vi "RX — NIRs.vi"() -> ()   [LabVIEW 2020]
panel:
  out "qC/N0":dbl[](array[numeric])
  out "Numeric":dbl
  out "Порог":dbl
  in  "Pлт":dbl=0.0001
  out "Array":cdb[][](array[numeric])
  out "Блок считывания":cdb[][](array[numeric])
  out "qC/N0 dB":dbl[](array[numeric])
  in  "Частота \nдискритезации":dbl=5000000.0 format="%#_13g"
  in  "Время \nнакопления":dbl=0.008 format="%#_13g"
  out "qC/N0":dbl
  out "dopEst":dbl
  out "codePhase":dbl
  in  "Целое число строк записанного файла":i32=50
  in  "Путь к записи сигнала":path=path "C:/Users/ira_1/OneDrive/Рабочий стол/samples.bin"
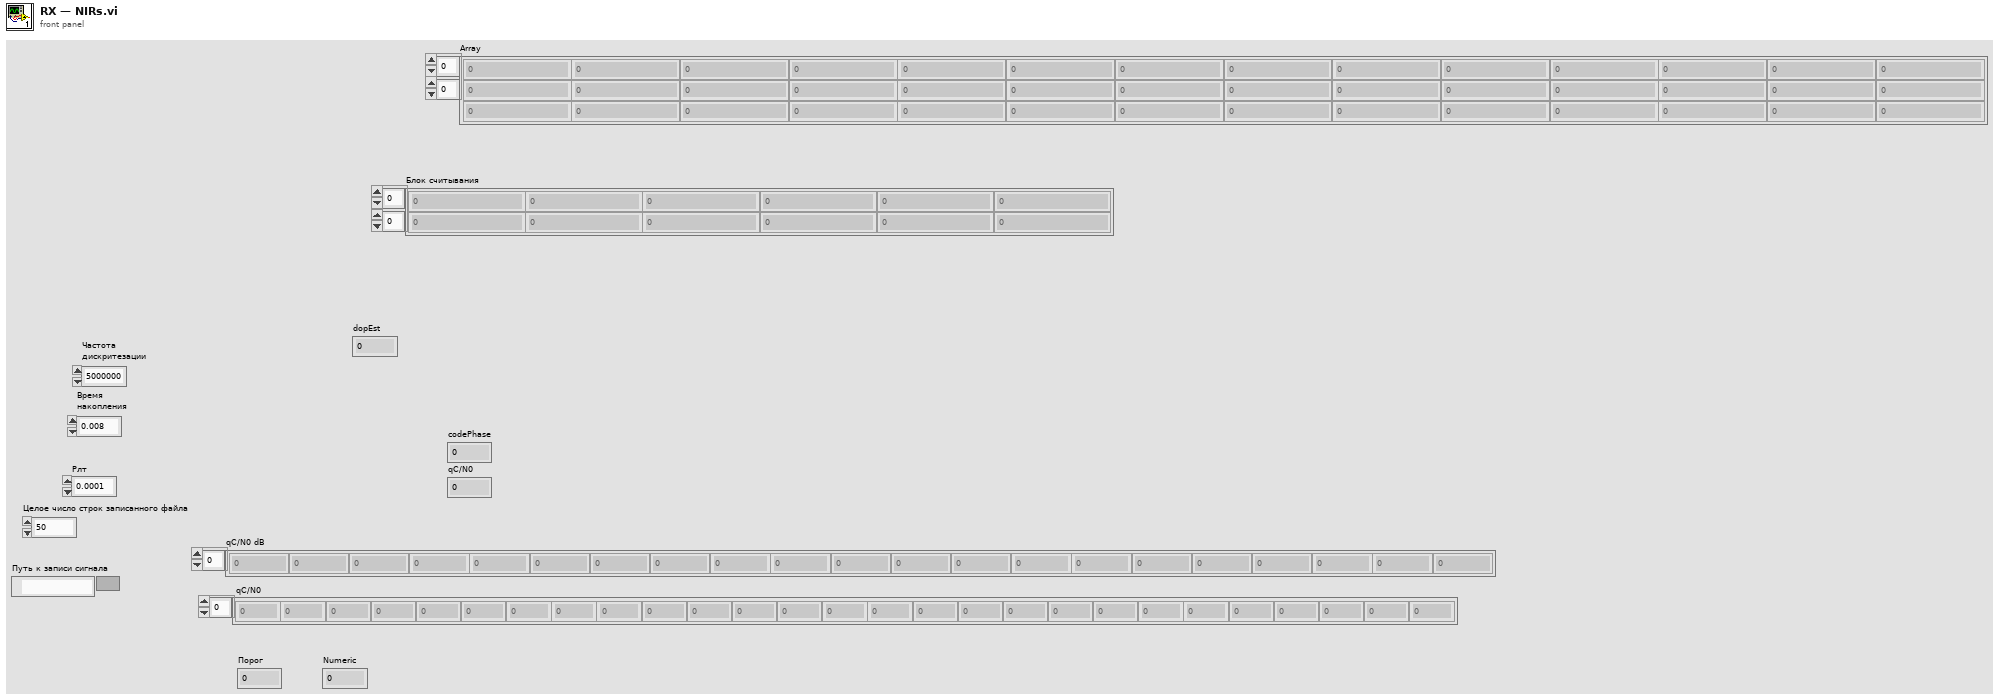
[diagram p1: front panel]
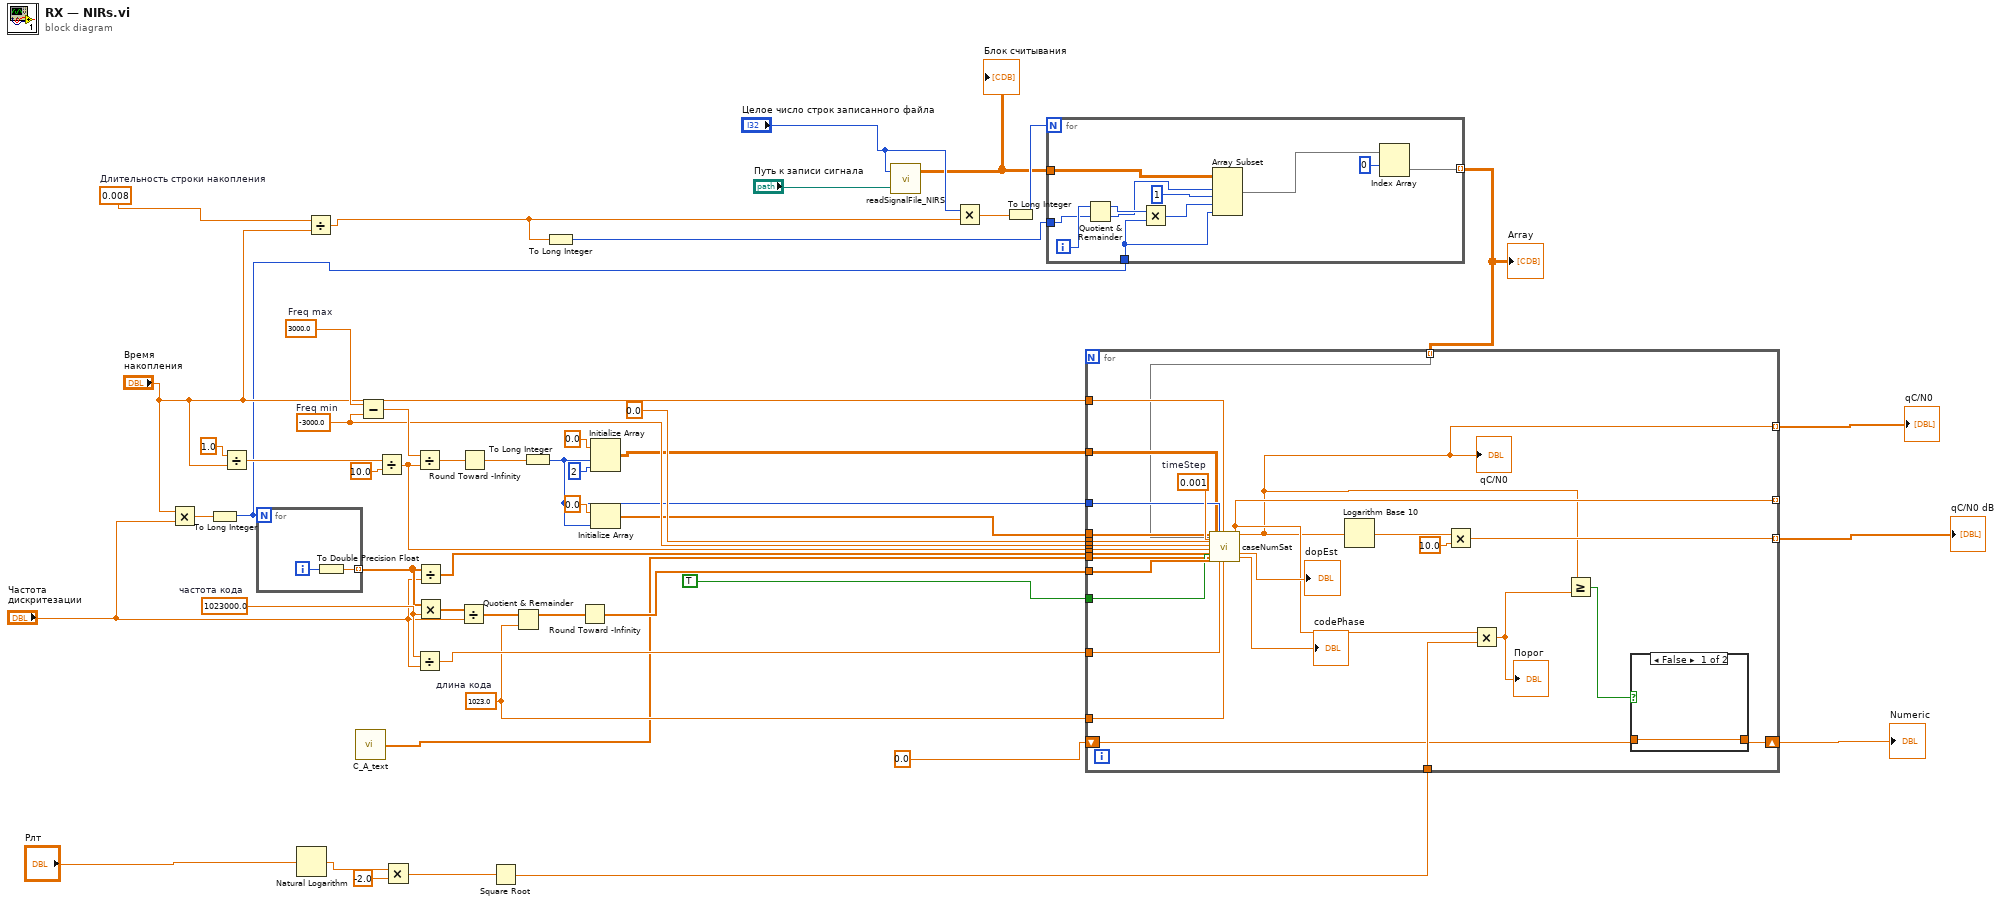
[diagram p0: block diagram]
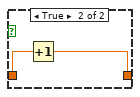
[diagram p2: hidden frame]
diagram:
  w20 = 0.008  # Длительность строки накопления
  w37 = -3000.0  # Freq min
  w43 = 3000.0  # Freq max
  w33 = 1023.0  # длина кода
  w35 = 1023000.0  # частота кода
  n1 = Multiply(x="Время \nнакопления", y="Частота \nдискритезации") -> (x*y=w21:dbl)
  n2 = To Long Integer(number=w21) -> (32bit integer=w14:i32)
  n3 = Divide(x=1.0, y="Время \nнакопления") -> (x/y=w39:dbl)
  n4 = for {
    N: w14 -> [_]
    tunnel: [w50] -> w25 mode=indexing
    i -> [w51]
    n5 = To Double Precision Float(number=w51) -> (double precision float=w50:dbl)
  }
  n6 = Natural Logarithm(1:"Pлт") -> (0:w11:dbl)
  n7 = Divide(x=w20, y="Время \nнакопления") -> (x/y=w16:dbl)
  n8 = call "C_A_text.vi"() -> ("array"=w23:dbl[])  [unwired: 2 in]
  n9 = Subtract(x=w43, y=w37) -> (x-y=w41:dbl)
  n10 = Divide(x=w39, y=10.0) -> (x/y=w36:dbl)
  n11 = Multiply(x=w11, y=-2.0) -> (x*y=w9:dbl)
  n12 = Divide(x=w41, y=w36) -> (x/y=w42:dbl)
  n13 = Divide(x=w35, y="Частота \nдискритезации") -> (x/y=w34:dbl)
  n14 = Divide(x=w25, y="Частота \nдискритезации") -> (x/y=w24:dbl[])
  n15 = Multiply(x=w25, y=w35) -> (x*y=w49:dbl[])
  n16 = Divide(x=w49, y="Частота \nдискритезации") -> (x/y=w48:dbl[])
  n17 = Round Toward -Infinity(1:w42) -> (0:w40:dbl)
  n18 = Square Root(x=w9) -> (sqrt(x)=w7:dbl)
  n19 = Quotient & Remainder(x=w48, y=w33) -> (x-y*floor(x/y)=w47:dbl[])  [unwired: 1 out]
  n20 = To Long Integer(number=w40) -> (32bit integer=w28:i32)
  n21 = To Long Integer(number=w16) -> (32bit integer=w15:i32)
  n22 = Round Toward -Infinity(1:w47) -> (0:w46:dbl[])
  n23 = Initialize Array(0.0 ("element"), w28, 2 ("dimension size")) -> (w27:dbl[][])
  n24 = Initialize Array(0.0 ("element"), w28) -> (w26:dbl[])
  n25 = call "readSignalFile_NIRS.vi"("Путь к записи сигнала"="Путь к записи сигнала", "Целое число строк записанного файла"="Целое число строк записанного файла") -> ("Array 2"=w2:cdb[][])  [unwired: 1 in]
  "Блок считывания" <- w2
  n26 = Multiply(x="Целое число строк записанного файла", y=w16) -> (x*y=w18:dbl)
  n27 = To Long Integer(number=w18) -> (32bit integer=w17:i32)
  n28 = for {
    N: w17 -> [_]
    tunnel: w2 -> [w62]
    tunnel: w15 -> [w60]
    tunnel: w14 -> [w58]
    tunnel: [w53] -> w13 mode=indexing
    i -> [w61]
    n29 = Quotient & Remainder(x=w61, y=w60) -> (x-y*floor(x/y)=w56:i32, floor(x/y)=w52:i32)
    n30 = Multiply(x=w56, y=w58) -> (x*y=w59:i32)
    n31 = Array Subset(array=w62, index (row)=w52, length (row)=1 ("length"), index (col)=w59, length (col)=w58) -> (w55:cdb[][])
    n32 = Index Array(array=w55, index (row)=0) -> (element=w53:cdb[])  [unwired: 1 in]
  }
  "Array" <- w13
  n33 = for {
    tunnel: w46 -> [w89]
    tunnel: 0.0 ("iFreq") -> [w88]
    tunnel: w37 -> [w87]
    tunnel: w36 -> [w86]
    tunnel: w34 -> [w85]
    tunnel: w33 -> [w84]
    tunnel: TRUE ("isThisNumTry") -> [w83]
    tunnel: w28 -> [w81]
    tunnel: w27 -> [w80]
    tunnel: w26 -> [w79]
    tunnel: w24 -> [w76]
    tunnel: "Время \nнакопления" -> [w73]
    tunnel: w23 -> [w72]
    tunnel: [w71] -> w8 mode=indexing
    tunnel: w13 -> [w70] mode=indexing
    tunnel: [w68] -> _ mode=indexing
    tunnel: w7 -> [w69]
    shift-right: [w64] -> w5
    shift-left: 0.0 -> [w65]
    tunnel: [w63] -> w1 mode=indexing
    w82 = 0.001  # timeStep
    n34 = call "caseNumSat.vi"("emptyVarCorrArr"=w79, "signalArrCDB"=w70, "iFreq"=w88, "Freq min"=w87, "Freq cell"=w86, "SampTimeArr"=w76, "PSPcodeL1C/A"=w72, "PSPcodeL1C/AIndex"=w89, "emptyCorrArr"=w80, "numCellFreq"=w81, "codeFreqDivAdcFreq"=w85, "timeAccumAcq"=w73, "codeLength"=w84, "timeStep"=w82, "isThisNumTry"=w83) -> ("mean"=w68:dbl, "cn0Est"=w63:dbl, "dopEst"=→"dopEst":dbl, "codePhase"=→"codePhase":dbl)  [unwired: 5 in, 4 out]
    "qC/N0" <- w63
    n35 = Logarithm Base 10(1:w63) -> (0:w75:dbl)
    n36 = Multiply(x=w75, y=10.0) -> (x*y=w71:dbl)
    n37 = Multiply(x=w68, y=w69) -> (x*y=w67:dbl)
    "Порог" <- w67
    n38 = Greater Or Equal?(x=w63, y=w67) -> (x >= y?=w66:bool)
    n39 = case shown="False" w66 {
      tunnel: w65 -> [w90 w92]
      tunnel: [w90 w91] -> w64
      frame False {
      }
      frame True {
        n40 = Increment(x=w92) -> (x+1=w91:dbl)
      }
    }
  }
  "qC/N0 dB" <- w8
  "Numeric" <- w5
  "qC/N0" <- w1
